vi "PE_program.vi"() -> ()   [LabVIEW 2015]
panel:
  in  "Tab Control":enum32{"Page 1", "Page 2"}(tab)
  out "Pulses 3":waveform(dbl)[](graph)
  in  "beta":dbl=0.5 format="%#_13g"
  in  "Offset":dbl(slide) scale=-1.0..1.0
  in  "PercentWidth":dbl(slide) scale=0.01..1.0
  in  "Number of sines":dbl(slide)=3.0 min=1.0 max=100.0 scale=1.0..20.0
  in  "Peak Finding Width":i32(slide)=3 min=3 max=100 step=1 scale=3.0..10.0
  out "XY Graph":cluster{dbl[], "Y":dbl[]}[](graph)
  out "Magnitude":waveform(dbl)(graph)
  out "Waveform Data":waveform(dbl)(graph)
  in  "milliseconds to wait":u32=1000
  in  "Stop Button":bool
  out "error out":errorcluster
  in  "error in (no error)":errorcluster
  out "VISA Refnum out":refnum<visa-resource-name>
  in  "Channels":u16[](array[ring])=[0] items=["Channel 1", "Channel 2", "Channel 3", "Channel 4", "Math 1", "Math 2", "Math 3", "Math 4", "Reference 1", "Reference 2", "Reference 3", "Reference 4"]
  in  "VISA Refnum in":refnum<visa-resource-name>
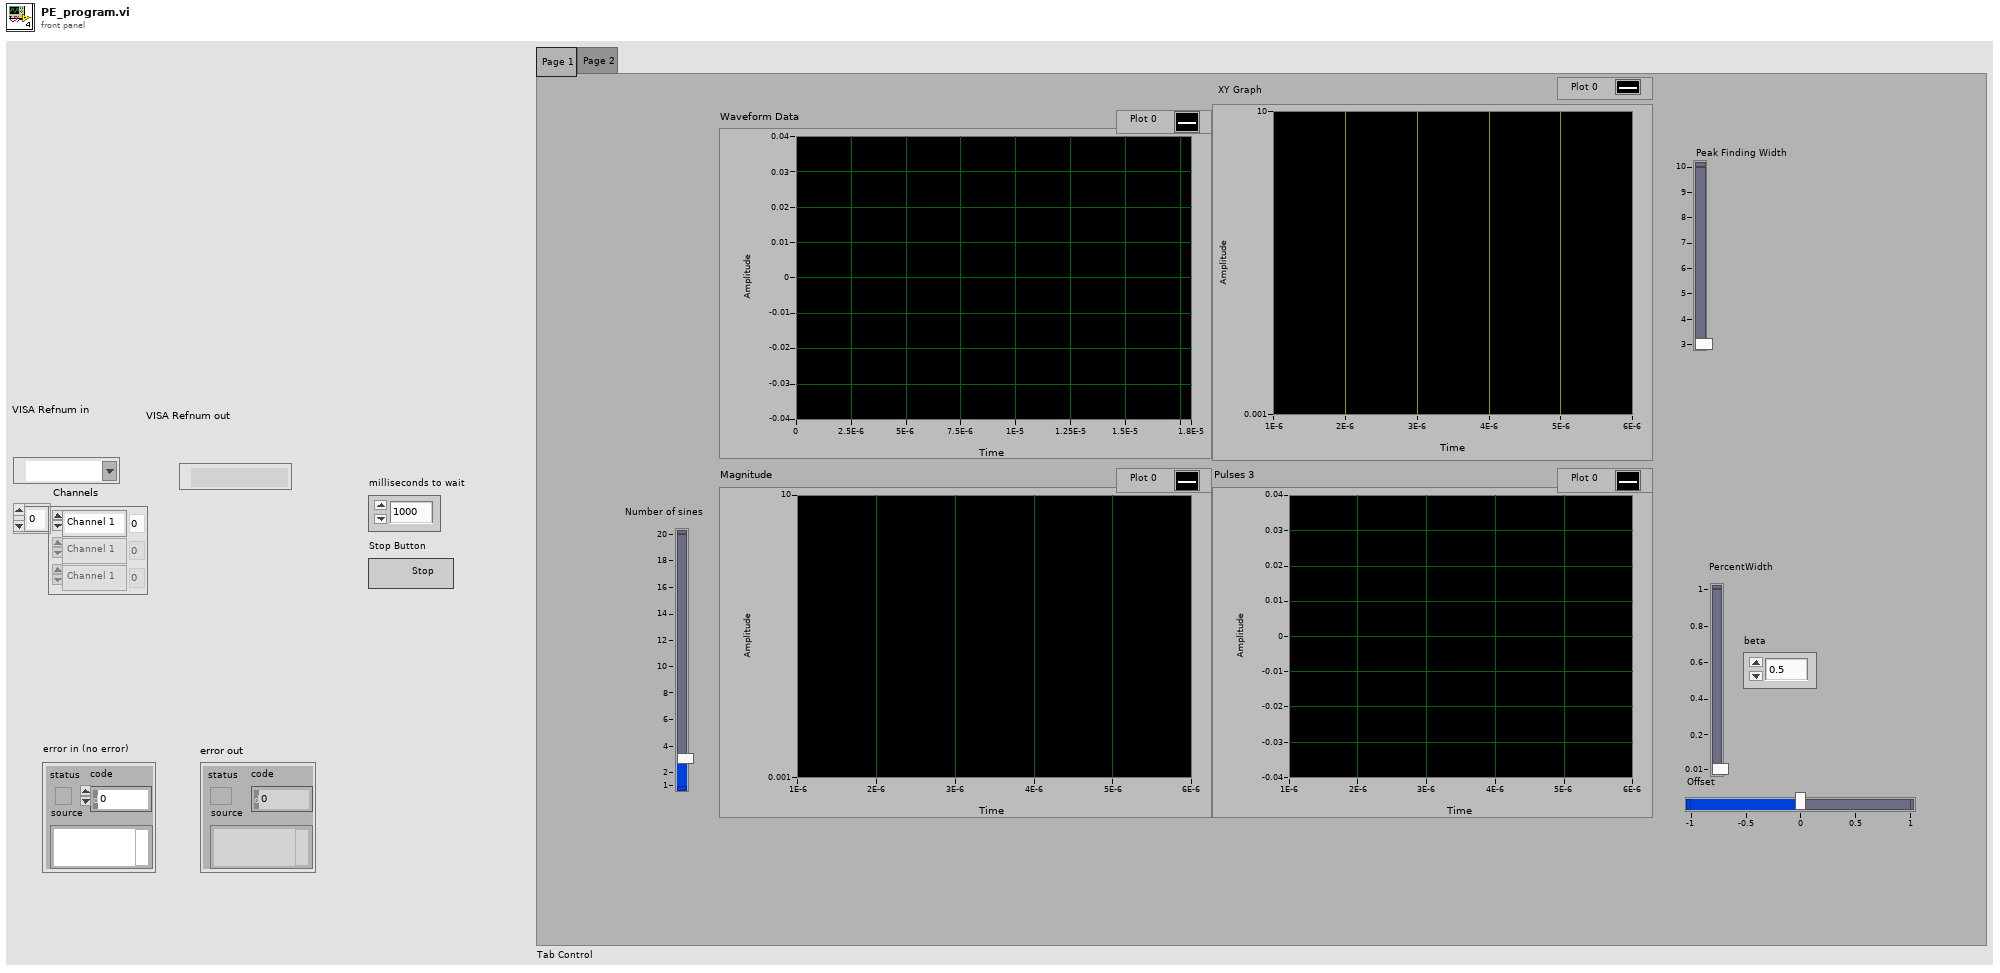
[diagram p1: front panel]
types:
  T1 = cluster{"Array":dbl[], "Best Exponential Fit":dbl[]}
  T2 = cluster{"Array":dbl[], "Best Exponential Fit":dbl[]}[]
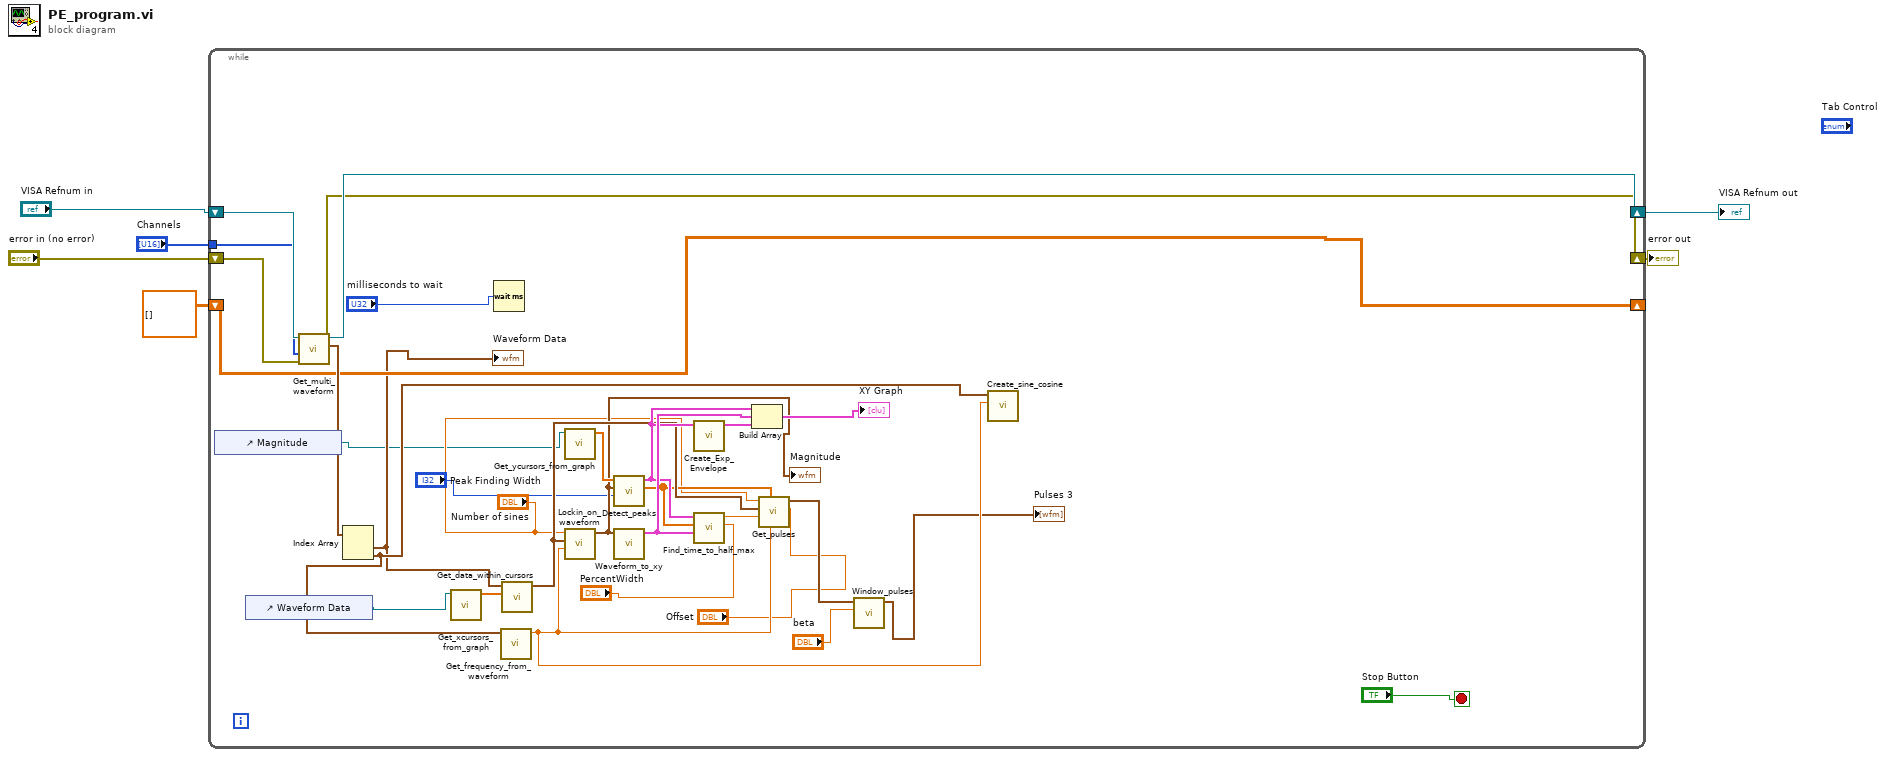
[diagram p0: block diagram]
diagram:
  n1 = while {
    tunnel: "Channels" -> [w36]
    shift-right: [w35] -> w4
    shift-left: "VISA Refnum in" -> [w37]
    shift-right: [w33] -> w2
    shift-left: "error in (no error)" -> [w34]
    shift-right: [w19] -> _
    shift-left: dbl[][] [] -> [w19]
    stop <- "Stop Button" stop-if-true
    n2 = control-ref of="Magnitude"() -> (w10:refnum<vi>)
    n3 = control-ref of="Waveform Data"() -> (w17:refnum<vi>)
    n4 = call "Get_multi_waveform.vi"("error in (no error)"=w34, "Channels"=w36, "VISA Refnum in"=w37) -> ("error out"=w33:errorcluster, "Waveform Data"=w32:waveform(dbl)[], "VISA Refnum out"=w35:refnum<visa-resource-name>)  [unwired: 6 in]
    n5 = Index Array(array=w32) -> (element #1=w18:waveform(dbl), element #2=w20:waveform(dbl))  [unwired: 2 in]
    "Waveform Data" <- w18
    n6 = call "Get_xcursors_from_graph.vi"("WaveformGraph in"=w17) -> ("Array"=w31:dbl[])  [unwired: 10 in]
    n7 = Wait (ms)(milliseconds to wait="milliseconds to wait") -> ()  [unwired: 1 out]
    n8 = call "Get_frequency_from_waveform.vi"("Waveform Data"=w20) -> ("Frequency"=w21:dbl)  [unwired: 9 in, 1 out]
    n9 = call "Get_data_within_cursors.vi"("Cursors"=w31, "Waveform Data"=w18) -> ("waveform out"=w23:waveform(dbl))  [unwired: 9 in]
    n10 = call "Get_ycursors_from_graph.vi"("WaveformGraph in"=w10) -> ("Array"=w30:dbl[])  [unwired: 10 in]
    n11 = call "Lockin_on_waveform.vi"("Frequency"=w21, "waveform in"=w23, "Number of Sines"="Number of sines") -> ("Magnitude"=w14:waveform(dbl))  [unwired: 7 in, 1 out]
    "Magnitude" <- w14
    n12 = call "Detect_peaks.vi"("width"="Peak Finding Width", "Magnitude"=w14, "Array"=w30) -> ("Locations"=w22:dbl[], "Peaks_xy"=w25:cluster{"Array":dbl[], "Amplitudes":dbl[]})  [unwired: 7 in]
    n13 = call "Waveform_to_xy.vi"("Magnitude"=w14) -> ("XY Pairs"=w26:cluster{"Array":dbl[], "Y":dbl[]})  [unwired: 10 in]
    n14 = call "Create_Exp_Envelope.vi"("Cluster in"=w25) -> ("Cluster out"=w29:T1)  [unwired: 10 in]
    n15 = call "Find_time_to_half_max.vi"("Slide"="PercentWidth", "XY_pairs_in"=w26, "Locations"=w22, "Peaks_xy_in"=w25) -> ("points_to_half_max"=w24:dbl)  [unwired: 7 in]
    n16 = Build Array(w25, w26, w29) -> (→"XY Graph":T2)
    n17 = call "Get_pulses.vi"("Offset"="Offset", "Frequency"=w21, "Locations"=w22, "points_to_half_max"=w24, "waveform in"=w23, "Number of sines"="Number of sines") -> ("Pulses"=w15:waveform(dbl)[])  [unwired: 5 in]
    n18 = call "Window_pulses.vi"("beta"="beta", "Pulses"=w15) -> ("Array"=→"Pulses 3":waveform(dbl)[])  [unwired: 9 in]
    n19 = call "Create_sine_cosine.vi"("Frequency"=w21, "Waveform Data"=w20) -> ()  [unwired: 8 in, 2 out]
  }
  "VISA Refnum out" <- w4
  "error out" <- w2
